vi "Query Active DUT Power Cycle State.vi"(8 "error in (no error)":errorcluster, 11 "VISA resource name":refnum<visa-resource-name>) -> (0 "error out":errorcluster, 2 "Power Cycle":i32, 3 "VISA resource name out":refnum<visa-resource-name>)   [LabVIEW 2020, in "Rohde&Schwarz CMXP Base.lvlib"]
doc: "Queries the state of the power cycle at the DUT.\n\nAttribute:\nRSCMXPBASE_ATTR_ACTIVE_DUT_POWER_CYCLE_STATE\n\nRemote-control command:\nFETCh:DUT:CONTrol:PCYCle:STATe?"
uses:
  <instrlib>/Rohde&Schwarz CMXP Base/Rohde&Schwarz CMXP Base.lvlib
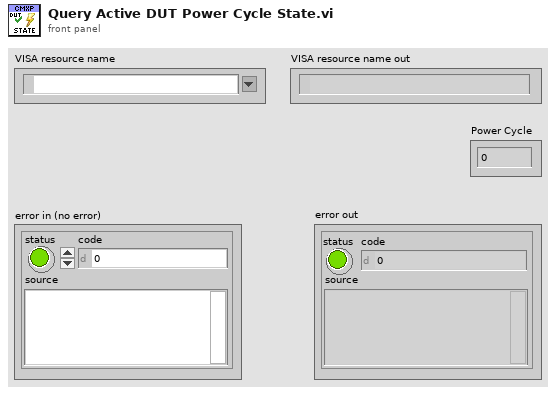
[diagram p1: front panel]
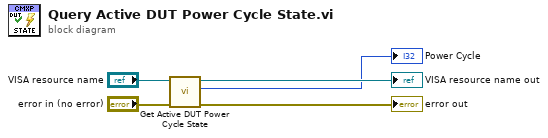
[diagram p0: block diagram]
diagram:
  n1 = call "Get Active DUT Power Cycle State"("error in (no error)"="error in (no error)", "instrument handle"="VISA resource name") -> ("error out"=→"error out":errorcluster, "Active DUT Power Cycle State"=→"Power Cycle":i32, "instrument handle out"=→"VISA resource name out":refnum<visa-resource-name>)  [unwired: 7 in]
